vi "SSL_Certification.vi"(8 "error in (no error)":errorcluster, 11 "DUT":string) -> (0 "error in (out)":errorcluster, 2 "Result":string)   [LabVIEW 2024, in "SSL_Certification.lvlib"]
doc: "This template is for the Queued Message Handler design pattern.\n\nThe Event Handling Loop generates messages based on user interface actions.\n\nThe Message Handling Loop processes messages generated by the Event Handling Loop, or by other messages. The messages are string values, so new messages can be added easily to the Message Cases case structure in the Message Handling Loop. Each message cluster can also provide an optional value for Message Data, which is a variant that can be converted to whatever message-specific data is required."
uses:
  SSL_Certification.lvlib
  support/Neoway_ctrl.ctl
  controls/Neoway UI Data.ctl
  PrivateControls/FGV_Queue_Control.ctl
  <vilib>/Utility/error.llb/Trim Whitespace One-Sided.vi
  <vilib>/Utility/error.llb/Error Cluster From Error Code.vi
  <vilib>/ErrorRing/Error Ring.xnode
  support/Message Queue/Neoway Message Queue.lvlib
  support/User Event - Stop/72-13360 User Event - Stop.lvlib
  Launcher/Launcher_DTU.lvlib
panel:
  out "Timer":i32
  in  "Neoway Flashing":T1
  in  "Config":string
  in  "Read_Res":bool
  in  "Read_Current":bool
  in  "Read_File":bool
  in  "Flash":bool
  out "queue name 2":string
  out "queue name":string
  out "Display <Replace Me>":string
  in  "Output":bool
  in  "Init_Neoway":bool
  in  "Exit":bool
  # "OKAY,River"
  # "These controls have associated \"Value Changed\" events configured in the Event Structure on the diagram.\n\nReplace them (and reconfigure the Event Structure) with the controls you need for your application."
  # "This template is for the Queued Message Handler design pattern.\n\nSee the block diagram for more information on how to use this template."
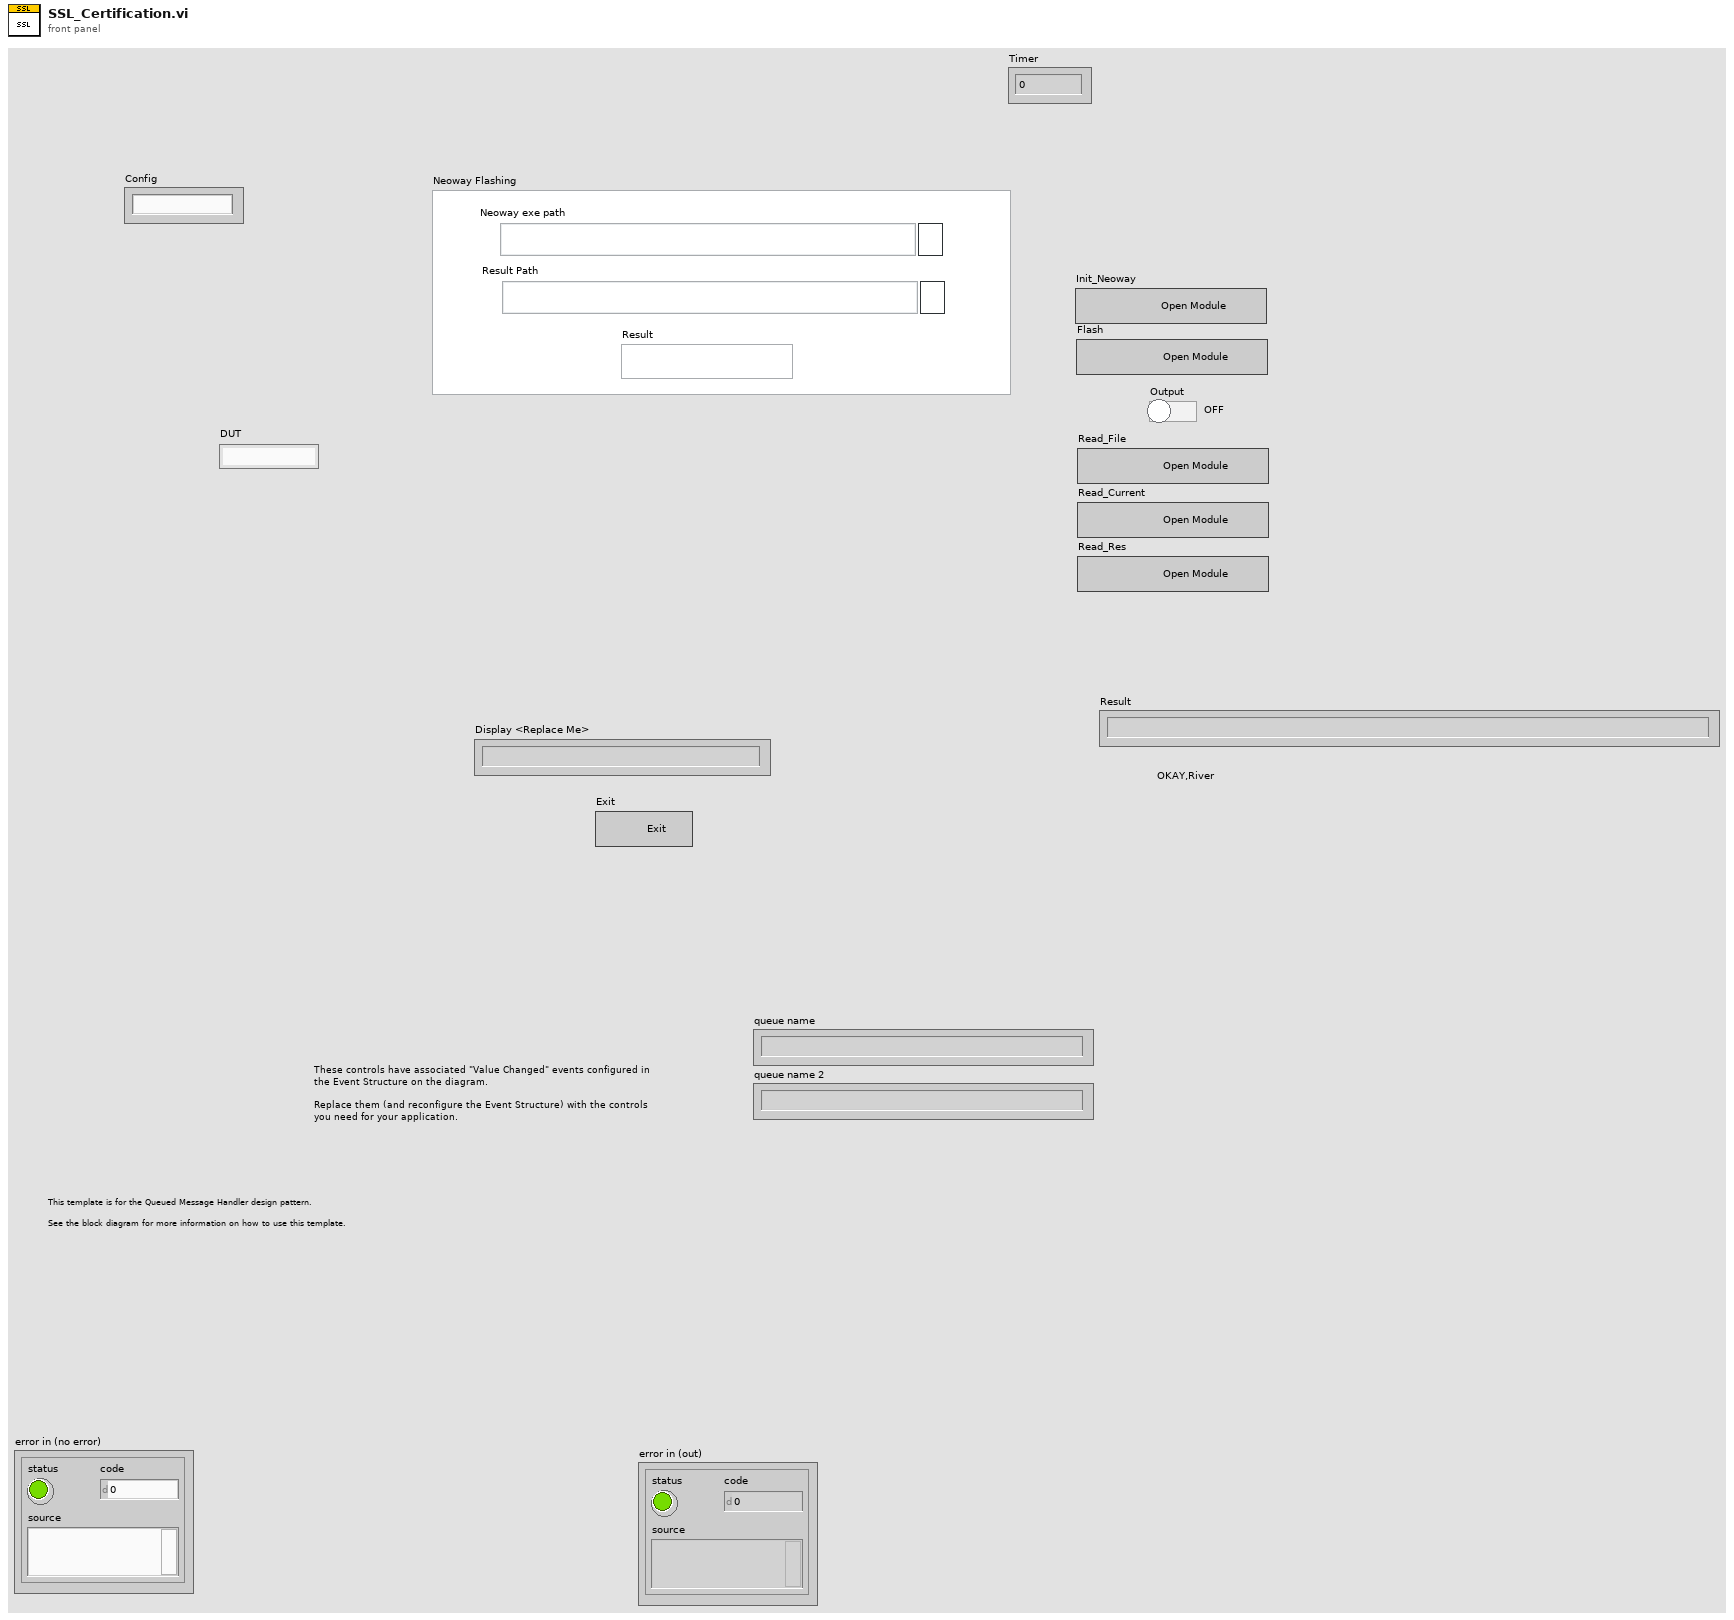
[diagram p1: front panel]
types:
  T1 = typedef "SSL_Certification.lvlib/Neoway_ctrl.ctl" = cluster{"Neoway exe path":path, "Result Path":path, "Result":string}
  T2 = typedef "SSL_Certification.lvlib/Neoway UI Data.ctl" = cluster{"DUT":string, "Neoway_Q":refnum<queue>, "notifier out":refnum<notifier>, "Config":string, "Neoway Flashing":T1, "Bat file path":path, "Exe path":string, "Flash path":string, "Result":string, "Timer":u32}
  T3 = typedef "SSL_Certification.lvlib/FGV_Queue_Control.ctl" = enum16{"Release", "Get", "Set"}
  T4 = typedef "SSL_Certification.lvlib/Neoway Message Queue.lvlib/All Message Queues.ctl" = cluster{"UI":refnum<queue>, "QSM":refnum<queue>}
  T5 = cluster{"Message":string, "Message Data":variant}
  T6 = enum16{"Read", "Write", "All_sections", "All_values", "Remove key&section"}
  T7 = enum16{"open", "replace", "create", "open or create", "replace or create", "replace or create with confirmation"}
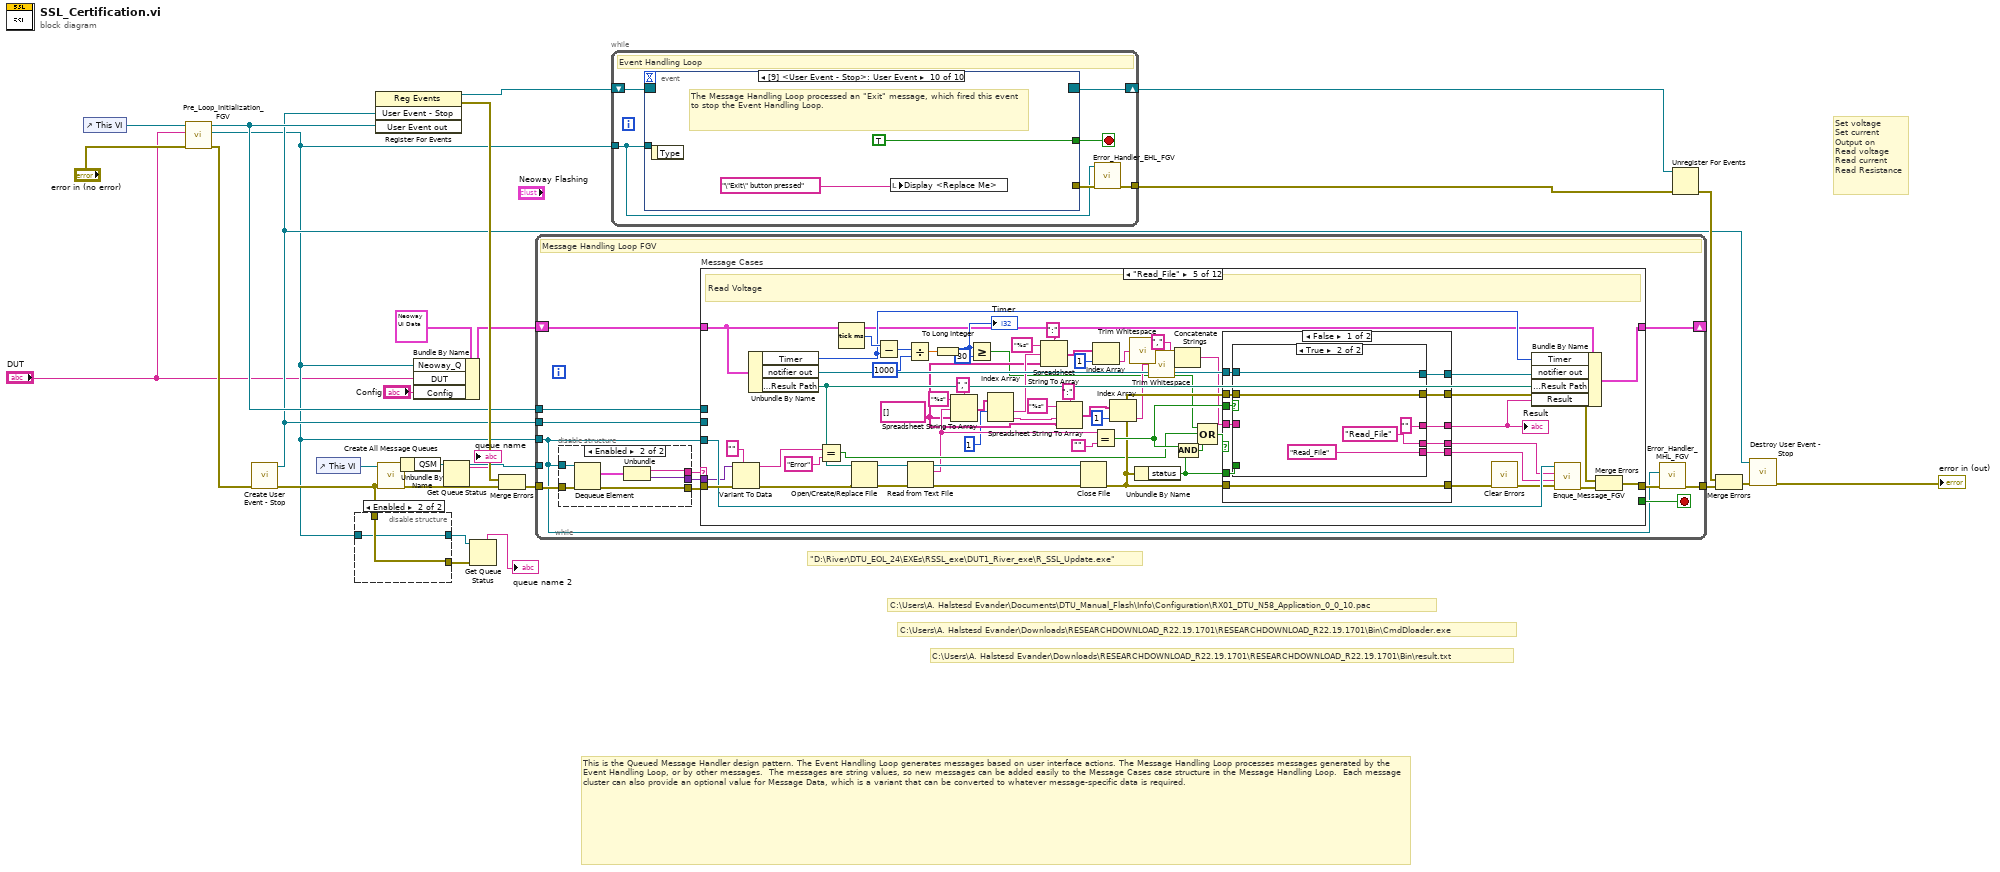
[diagram p0: block diagram]
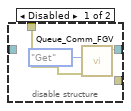
[diagram p2: hidden frame]
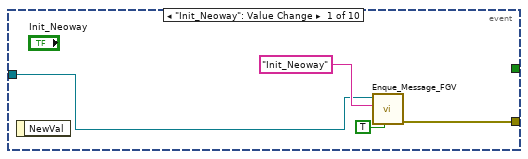
[diagram p3: hidden frame]
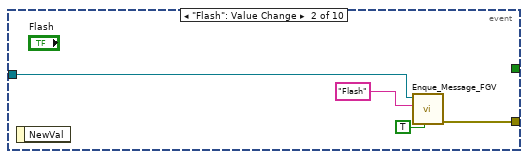
[diagram p4: hidden frame]
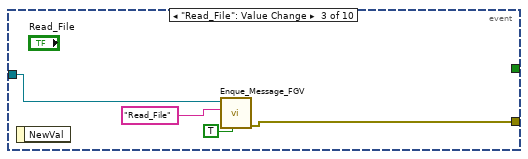
[diagram p5: hidden frame]
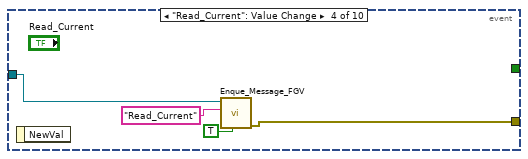
[diagram p6: hidden frame]
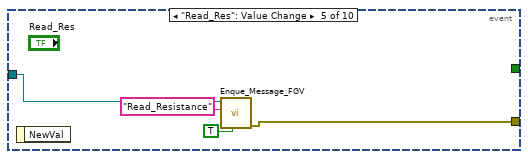
[diagram p7: hidden frame]
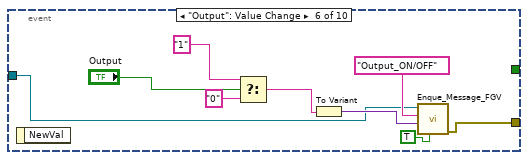
[diagram p8: hidden frame]
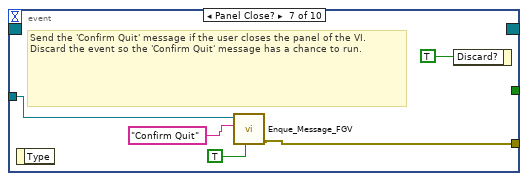
[diagram p9: hidden frame]
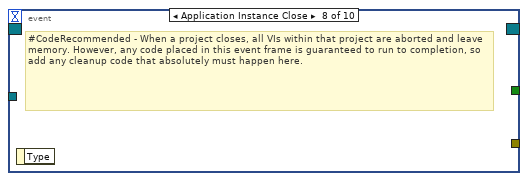
[diagram p10: hidden frame]
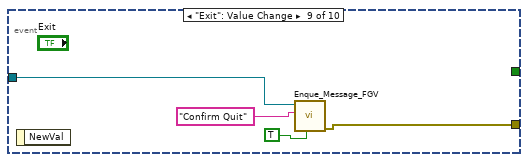
[diagram p11: hidden frame]
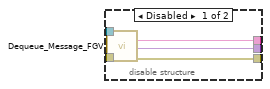
[diagram p12: hidden frame]
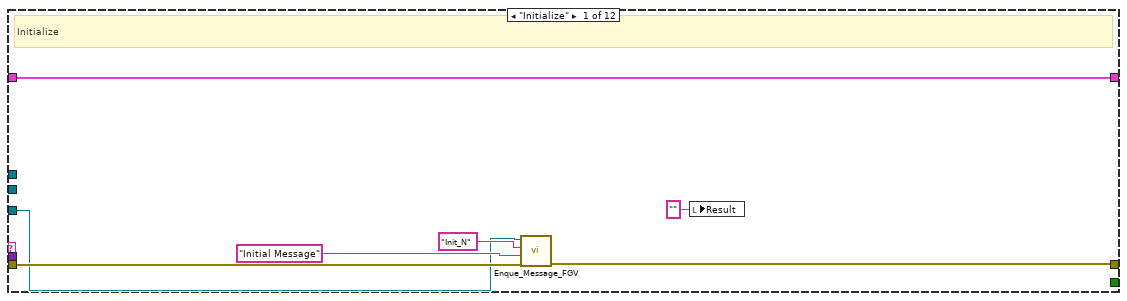
[diagram p13: hidden frame]
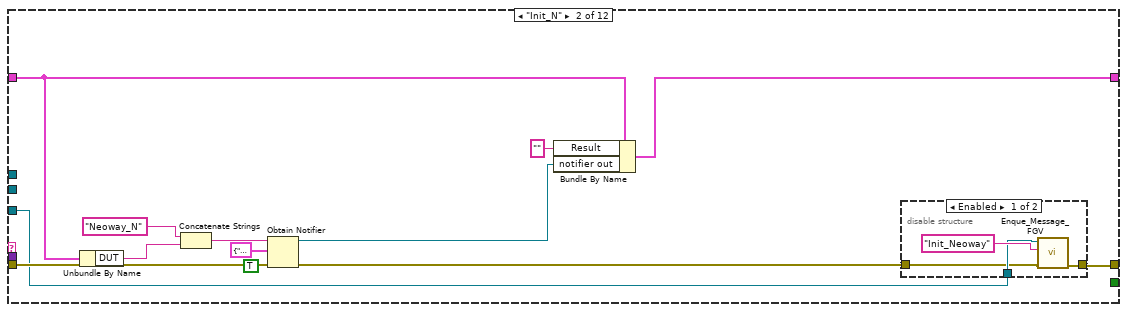
[diagram p14: hidden frame]
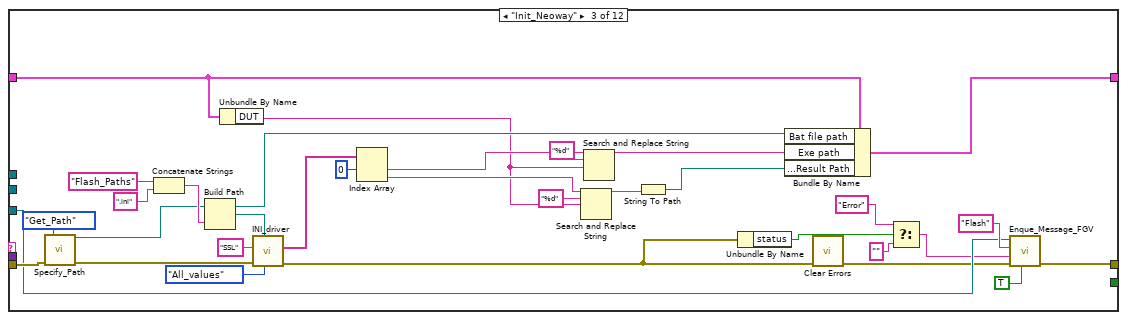
[diagram p16: hidden frame]
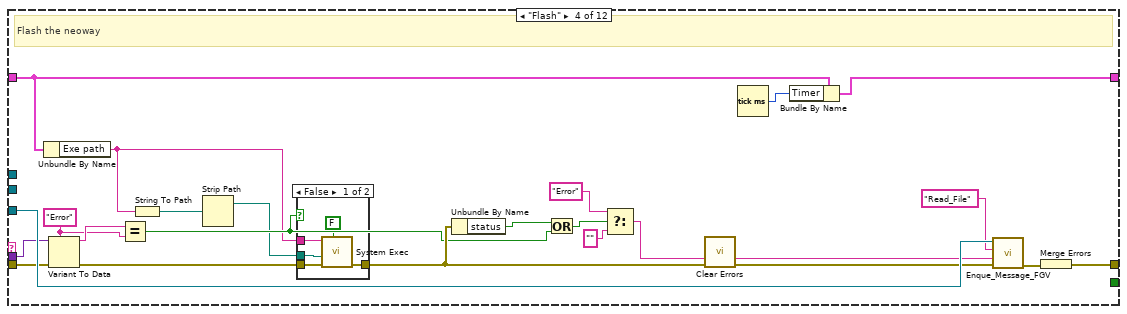
[diagram p17: hidden frame]
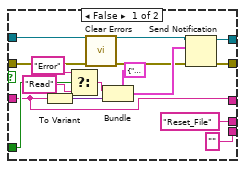
[diagram p19: hidden frame]
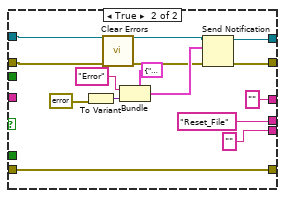
[diagram p20: hidden frame]
diagram:
  # "\"D:\\River\\DTU_EOL_24\\EXEs\\RSSL_exe\\DUT1_River_exe\\R_SSL_Update.exe\""
  # "C:\\Users\\A. Halstesd Evander\\Downloads\\RESEARCHDOWNLOAD_R22.19.1701\\RESEARCHDOWNLOAD_R22.19.1701\\Bin\\result.txt"
  # "C:\\Users\\A. Halstesd Evander\\Downloads\\RESEARCHDOWNLOAD_R22.19.1701\\RESEARCHDOWNLOAD_R22.19.1701\\Bin\\CmdDloader.exe"
  # "C:\\Users\\A. Halstesd Evander\\Documents\\DTU_Manual_Flash\\Info\\Configuration\\RX01_DTU_N58_Application_0_0_10.pac"
  # "Set voltage\nSet current\nOutput on\nRead voltage \nRead current\nRead Resistance"
  # "This is the Queued Message Handler design pattern. The Event Handling Loop generates messages based on user interface actions. The Message Handling Loop processes messages generated by the Event Handling Loop, or by other messages.  The messages are string values, so new messages can be added easily to the Message Cases case structure in the Message Handling Loop.  Each message cluster can also provide an optional value for Message Data, which is a variant that can be converted to whatever message-specific data is required."
  n1 = control-ref of="This VI"() -> (w17:refnum<vi>)
  n2 = call "Pre_Loop_Initialization_FGV.vi"("error in (no error)"="error in (no error)", "DUT"="DUT", "VI in"=w17) -> ("error out"=w15:errorcluster, "queue out"=w3:refnum<queue>, "User Event out"=w7:refnum<user-event>)  [unwired: 6 in]
  n3 = call "Create User Event - Stop.vi"("error in (no error)"=w15) -> ("error out"=w10:errorcluster, "User Event - Stop"=w6:refnum<user-event>)  [unwired: 9 in]
  n4 = control-ref of="This VI"() -> (w13:refnum<vi>)
  n5 = disable-structure shown="Enabled" {
    disable-tunnel: w10 -> [w32 w34]
    disable-tunnel: [w30 w33] -> w9
    disable-tunnel: [_ w34] -> w5
    disable-tunnel: w3 -> [_ w33]
    frame Disabled {
      n6 = call "Queue_Comm_FGV.vi"("error in (no error)"=w32, "Enum"=FGV_Queue_Control."Get") -> ("queue Out"=w30:refnum<queue>)  [unwired: 8 in, 1 out]
    }
    frame Enabled {
    }
  }
  n7 = register-events(w6, w7) -> (reference out=w20:refnum<event-registration>, error out=w18:errorcluster)  [unwired: 2 in]
  n8 = call "Create All Message Queues.vi"("error in (no error)"=w10, "This VI"=w13) -> ("error out"=w29:errorcluster, "Message Queues out"=w28:T4)  [unwired: 8 in]
  n9 = Unbundle By Name(w28) -> ("QSM"=w26:refnum<queue>)
  n10 = Bundle By Name(cluster=T2 {"DUT"="", "Neoway_Q"=refnum, "notifier out"=refnum, "Config"="", "Neoway Flashing"={"Neoway exe path"=path "", "Result Path"=path "", "Result"=""}, "Bat file path"=path "", "Exe path"="", "Flash path"="", "Result"="", "Timer"=0} ("Data Cluster"), "Neoway_Q"=w3, "DUT"="DUT", "Config"="Config") -> (w4:T2)
  n11 = Get Queue Status(queue=w26) -> (queue out=w12:refnum<queue>, queue name=→"queue name":string)  [unwired: 2 in, 6 out]
  n12 = Get Queue Status(queue=w9, error in (no error)=w5) -> (queue name=→"queue name 2":string)  [unwired: 1 in, 7 out]
  n13 = Merge Errors(w18, w29) -> (w19:errorcluster)
  n14 = while {
    tunnel: w12 -> [_]
    shift-right: [w45] -> _
    shift-left: w4 -> [w46]
    tunnel: w7 -> [w43]
    tunnel: w19 -> [w42]
    tunnel: [w37] -> w27
    tunnel: w6 -> [w36]
    tunnel: w3 -> [w35]
    stop <- w44 stop-if-true
    # "Message Handling Loop FGV"
    n15 = disable-structure shown="Enabled" {
      disable-tunnel: w42 -> [w50 w56]
      disable-tunnel: [w49 w54] -> w41
      disable-tunnel: [w48 w51] -> w40
      disable-tunnel: [w47 w52] -> w39
      disable-tunnel: w35 -> [_ w55]
      frame Disabled {
        n16 = call "Dequeue_Message_FGV.vi"("error in (no error)"=w50) -> ("error out"=w49:errorcluster, "Message Data"=w48:variant, "Message"=w47:string)  [unwired: 8 in]
      }
      frame Enabled {
        n17 = Dequeue Element(queue=w55, error in (no error)=w56) -> (element=w53:T5, error out=w54:errorcluster)  [unwired: 1 in, 2 out]
        n18 = Unbundle(w53) -> ("Message"=w52:string, "Message Data"=w51:variant)
      }
    }
    n19 = case "Message Cases" shown="\"Read_File\"" w39 {
      selector: w39 -> [_ _ _ _ _ _ _ _ _ _ _ w313]
      tunnel: w41 -> [w59 w76 w113 w133 w203 w263 w273 w282 w291 w296 w304 _]
      tunnel: [w62 w65 w89 w136 w199 w250 w265 w280 w293 w294 w297 w314] -> w38
      tunnel: w46 -> [w63 w74 w98 w132 w143 w262 w274 w281 w288 w295 w299 w315]
      tunnel: [w63 w69 w103 w115 w201 w262 w274 w281 w288 w295 w299 w315] -> w45
      tunnel: [_ _ _ _ _ _ _ _ _ _ TRUE _] -> w44
      tunnel: w40 -> [_ _ _ w123 w198 _ w272 _ _ _ w306 _]
      tunnel: w43 -> [_ _ _ _ _ _ _ _ _ _ w307 _]
      tunnel: w36 -> [_ _ _ _ _ _ _ _ _ _ w302 _]
      tunnel: w35 -> [w58 w67 w88 w134 w200 w249 w264 w275 w286 _ w298 _]
      frame "Initialize" {
        # "Initialize"
        n20 = call "Enque_Message_FGV.vi"("error in (no error)"=w59, "Message Data"="Initial Message" ("Initial Message"), "Message"="Init_N", "queue in"=w58) -> ("error out"=w62:errorcluster)  [unwired: 7 in]
        n21 = local write "Result"("" ("Result")) -> ()
      }
      frame "Init_N" {
        n22 = Unbundle By Name(w74) -> ("DUT"=w73:string)
        n23 = Concatenate Strings("Neoway_N", w73) -> (w72:string)
        n24 = Obtain Notifier(name (unnamed)=w72, notification data type=T5 {"Message"="", "Message Data"=variant} ("notification"), create if not found? (T)=TRUE, error in (no error)=w76) -> (notifier out=w68:refnum<notifier>, error out=w66:errorcluster)  [unwired: 1 out]
        n25 = Bundle By Name(cluster=w74, "Result"="", "notifier out"=w68) -> (w69:T2)
        n26 = disable-structure shown="Enabled" {
          disable-tunnel: w67 -> [w79 _]
          disable-tunnel: w66 -> [w78 w81]
          disable-tunnel: [w77 w81] -> w65
          frame Enabled {
            n27 = call "Enque_Message_FGV.vi"("error in (no error)"=w78, "Message"="Init_Neoway", "queue in"=w79) -> ("error out"=w77:errorcluster)  [unwired: 8 in]
          }
          frame Disabled {
          }
        }
      }
      frame "Init_Neoway" {
        n28 = call "Specify_Path.vi"("Path_Enum"=enum16{"Find_Path", "Get_Path"}."Get_Path", "error in (no error)"=w113) -> ("Configurations"=w101:path, "error out"=w108:errorcluster)  [unwired: 6 in, 6 out]
        n29 = Concatenate Strings("Flash_Paths" ("string"), ".ini" ("string")) -> (w110:string)
        n30 = Build Path(base path=w101, name or relative path=w110) -> (appended path=w109:path)
        n31 = Unbundle By Name(w98) -> ("DUT"=w94:string)
        n32 = call "INI_driver.vi"("Enum"=T6."All_values", "instrument file path"=w109, "error in (no error)"=w108, "Section"="SSL") -> ("error out"=w84:errorcluster, "Values out"=w106:string[])  [unwired: 4 in, 2 out]
        n33 = Index Array(array=w106, index #1=0 ("index")) -> (element #1=w100:string, element #2=w95:string)  [unwired: 1 in]
        n34 = Search and Replace String(input string=w95, search string="%d", replace string=w94) -> (result string=w93:string)  [unwired: 5 in, 3 out]
        n35 = Search and Replace String(input string=w100, search string="%d", replace string=w94) -> (result string=w97:string)  [unwired: 5 in, 3 out]
        n36 = String To Path(string=w93) -> (path=w92:path)
        n37 = Unbundle By Name(w84) -> ("status"=w86:bool)
        n38 = Bundle By Name(cluster=w98, "Bat file path"=w101, "Exe path"=w97, "Neoway Flashing.Result Path"=w92) -> (w103:T2)
        n39 = call <vilib>:"Clear Errors.vi"("error in (no error)"=w84) -> ("error out"=w82:errorcluster)  [unwired: 5 in, 1 out]
        n40 = Select(t="Error" ("\"Do Something\" button pressed"), s=w86, f="" ("\"Do Something\" button pressed")) -> (s? t:f=w83:string)
        n41 = call "Enque_Message_FGV.vi"("Priority"=TRUE ("Priority Message? (F)"), "error in (no error)"=w82, "Message Data"=w83, "Message"="Flash", "queue in"=w88) -> ("error out"=w89:errorcluster)  [unwired: 6 in]
      }
      frame "Flash" {
        w120 = "Error" ("Message")
        # "Flash the neoway"
        n42 = Unbundle By Name(w132) -> ("Exe path"=w118:string)
        n43 = Variant To Data(error in=w133, type=w120, Variant=w123) -> (data=w121:string, error out=w124:errorcluster)
        n44 = Equal?(x=w121, y=w120) -> (x = y?=w119:bool)
        n45 = String To Path(string=w118) -> (path=w117:path)
        n46 = Strip Path(path=w117) -> (stripped path=w116:path)  [unwired: 1 out]
        n47 = case shown="False" w119 {
          tunnel: w118 -> [w141 _]
          tunnel: [w140 w142] -> w131
          tunnel: w124 -> [w139 w142]
          tunnel: w116 -> [w137 _]
          frame False {
            n48 = call <vilib>:"System Exec.vi"("wait until completion? (T)"=FALSE, "error in (no error)"=w139, "working directory"=w137, "command line"=w141) -> ("error out"=w140:errorcluster)  [unwired: 4 in, 3 out]
          }
          frame True {
          }
        }
        n49 = Unbundle By Name(w131) -> ("status"=w128:bool)
        n50 = Or(x=w128, y=w119) -> (x .or. y?=w122:bool)
        n51 = Select(t="Error" ("\"Do Something\" button pressed"), s=w122, f="" ("\"Do Something\" button pressed")) -> (s? t:f=w126:string)
        n52 = call <vilib>:"Clear Errors.vi"("error in (no error)"=w131) -> ("error out"=w125:errorcluster)  [unwired: 5 in, 1 out]
        n53 = Tick Count (ms)() -> (millisecond timer value=w114:u32)
        n54 = Bundle By Name(cluster=w132, "Timer"=w114) -> (w115:T2)
        n55 = call "Enque_Message_FGV.vi"("error in (no error)"=w125, "Message Data"=w126, "Message"="Read_File", "queue in"=w134) -> ("error out"=w135:errorcluster)  [unwired: 7 in]
        n56 = Merge Errors(w135) -> (w136:errorcluster)
      }
      frame "Read_File" {
        w165 = string[] []
        # "Read Voltage"
        n57 = Variant To Data(error in=w203, type="", Variant=w198) -> (data=w195:string, error out=w194:errorcluster)
        n58 = Unbundle By Name(w143) -> ("Timer"=w149:u32, "notifier out"=w185:refnum<notifier>, "Neoway Flashing.Result Path"=w188:path)
        n59 = Equal?(x=w195, y="Error" ("\"Do Something\" button pressed")) -> (x = y?=w177:bool)
        n60 = Tick Count (ms)() -> (millisecond timer value=w155:u32)
        n61 = Open/Create/Replace File(file path (use dialog)=w188, error in=w194) -> (refnum out=w191:refnum<file>, error out=w193:errorcluster)  [unwired: 4 in, 1 out]
        n62 = Subtract(x=w155, y=w149) -> (x-y=w154:u32)
        n63 = Divide(x=w154, y=u32 1000) -> (x/y=w152:dbl)
        n64 = Read from Text File(file (use dialog)=w191, error in=w193) -> (refnum out=w189:refnum<file>, text=w174:string, error out=w192:errorcluster)  [unwired: 2 in, 1 out]
        n65 = To Long Integer(number=w152) -> (32bit integer=w148:i32)
        "Timer" <- w148
        n66 = Spreadsheet String To Array(delimiter (Tab)=",", format string="%s", spreadsheet string=w174, array type (2D Dbl)=w165) -> (array=w171:string[])
        n67 = Greater Or Equal?(x=w148, y=30) -> (x >= y?=w150:bool)
        n68 = Index Array(array=w171, index #1=1 ("index")) -> (element #1=w166:string, element #2=w164:string)  [unwired: 1 in]
        n69 = Spreadsheet String To Array(delimiter (Tab)=":", format string="%s", spreadsheet string=w166, array type (2D Dbl)=w165) -> (array=w163:string[])
        n70 = Spreadsheet String To Array(delimiter (Tab)=":", format string="%s", spreadsheet string=w164, array type (2D Dbl)=w165) -> (array=w160:string[])
        n71 = Close File(refnum=w189, error in=w192) -> (error out=w179:errorcluster)  [unwired: 1 out]
        n72 = Equal?(x=w174, y="") -> (x = y?=w182:bool)
        n73 = Index Array(array=w163, index=1) -> (element=w159:string)
        n74 = Index Array(array=w160, index=1) -> (element=w157:string)
        n75 = call <vilib>:"Trim Whitespace.vi"("string"=w159) -> ("trimmed string"=w145:string)  [unwired: 1 in]
        n76 = Unbundle By Name(w179) -> ("status"=w183:bool)
        n77 = call <vilib>:"Trim Whitespace.vi"("string"=w157) -> ("trimmed string"=w144:string)  [unwired: 1 in]
        n78 = Concatenate Strings(w145, "," ("string"), w144) -> (w156:string)
        n79 = Compound Arithmetic op=AND(w182, w183) -> (w176:bool)
        n80 = Compound Arithmetic op=OR(w150, w177, w176) -> (w175:bool)
        n81 = case shown="False" w175 {
          tunnel: w179 -> [w214 w240]
          tunnel: [w213 w241] -> w186
          tunnel: w185 -> [w212 w243]
          tunnel: [w211 w242] -> w184
          tunnel: w156 -> [w210 _]
          tunnel: w183 -> [w209 _]
          tunnel: w182 -> [w208 _]
          tunnel: [w207 "Reset_File" ("Message")] -> w181
          tunnel: [w206 "" ("\"Do Something\" button pressed")] -> w180
          tunnel: w179 -> [w205 w248]
          tunnel: [w205 w248] -> w178
          tunnel: [w204 ""] -> w147
          frame False {
            n82 = case shown="True" w208 {
              tunnel: w214 -> [w223 w234]
              tunnel: [w221 w234] -> w213
              tunnel: w212 -> [w220 w233]
              tunnel: [w219 w233] -> w211
              tunnel: w210 -> [w215 _]
              tunnel: w209 -> [w218 _]
              tunnel: ["Reset_File" ("Message") "Read_File" ("Message")] -> w207
              tunnel: ["" ("\"Do Something\" button pressed") "Read_File" ("\"Do Something\" button pressed")] -> w206
              tunnel: [w215 ""] -> w204
              frame False {
                n83 = To Variant(anything=w215) -> (Variant=w228:variant)
                n84 = Select(t="Error" ("f"), s=w218, f="Read" ("Message")) -> (s? t:f=w229:string)
                n85 = call <vilib>:"Clear Errors.vi"("error in (no error)"=w223) -> ("error out"=w222:errorcluster)  [unwired: 5 in, 1 out]
                n86 = Bundle(cluster=T5 {"Message"="", "Message Data"=variant} ("notification"), "Message"=w229, "Message Data"=w228) -> (w227:T5)
                n87 = Send Notification(notification=w227, notifier=w220, error in (no error)=w222) -> (notifier out=w219:refnum<notifier>, error out=w221:errorcluster)
              }
              frame True {
              }
            }
          }
          frame True {
            n88 = To Variant(anything=errorcluster {"status"=TRUE, "code"=0, "source"="Error at N58 Flashing"} ("error constant")) -> (Variant=w247:variant)
            n89 = call <vilib>:"Clear Errors.vi"("error in (no error)"=w240) -> ("error out"=w244:errorcluster)  [unwired: 5 in, 1 out]
            n90 = Bundle(cluster=T5 {"Message"="", "Message Data"=variant} ("notification"), "Message"="Error" ("f"), "Message Data"=w247) -> (w246:T5)
            n91 = Send Notification(notification=w246, notifier=w243, error in (no error)=w244) -> (notifier out=w242:refnum<notifier>, error out=w241:errorcluster)
          }
        }
        "Result" <- w147
        n92 = call <vilib>:"Clear Errors.vi"("error in (no error)"=w178) -> ("error out"=w187:errorcluster)  [unwired: 5 in, 1 out]
        n93 = Bundle By Name(cluster=w143, "Timer"=w149, "notifier out"=w184, "Neoway Flashing.Result Path"=w188, "Result"=w147) -> (w201:T2)
        n94 = call "Enque_Message_FGV.vi"("error in (no error)"=w187, "Message Data"=w180, "Message"=w181, "queue in"=w200) -> ("error out"=w202:errorcluster)  [unwired: 7 in]
        n95 = Merge Errors(w186, w202) -> (w199:errorcluster)
      }
      frame "Reset_File" {
        n96 = Unbundle By Name(w262) -> ("Neoway Flashing.Result Path"=w260:path)  [unwired: 1 out]
        n97 = Open/Create/Replace File(file path (use dialog)=w260, error in=w263, operation (0:open)=T7."replace") -> (refnum out=w257:refnum<file>, error out=w261:errorcluster)  [unwired: 3 in, 1 out]
        n98 = Read from Text File(file (use dialog)=w257, error in=w261) -> (refnum out=w254:refnum<file>, text=w255:string, error out=w258:errorcluster)  [unwired: 2 in, 1 out]
        n99 = Equal?(x=w255, y="") -> ()  [unwired: 1 out]
        n100 = Close File(refnum=w254, error in=w258) -> (error out=w251:errorcluster)  [unwired: 1 out]
        n101 = call "Enque_Message_FGV.vi"("error in (no error)"=w251, "Message Data"="Resetted Flash file" ("\"Do Something\" button pressed"), "Message"="Update Display", "queue in"=w249) -> ("error out"=w250:errorcluster)  [unwired: 7 in]
      }
      frame "Update Display" {
        # "#CodeRecommended - If you wish to decouple the Message Handling Loop from your user interface, consider creating User Events (like the \"Stop\" event in this VI) to message the Event Handling Loop whenever the user interface needs updating."
        # "Update Display - Convert the message data to a string to display in the Data Display indicator."
        n102 = Variant To Data(error in=w273, type="", Variant=w272) -> (data=→"Display <Replace Me>":string, error out=w270:errorcluster)
        n103 = call <vilib>:"Clear Errors.vi"("error in (no error)"=w270) -> ("error out"=w268:errorcluster)  [unwired: 5 in, 1 out]
        n104 = Merge Errors(w268) -> (w266:errorcluster)
        n105 = call "Enque_Message_FGV.vi"("error in (no error)"=w266, "Message"="Confirm Quit", "queue in"=w264) -> ("error out"=w265:errorcluster)  [unwired: 8 in]
      }
      frame "Error" {
        # "Error - Display an error dialog. This message is sent by the \"Error Handler\" VIs at the end of other loops in this application."
        n106 = call <vilib>:"Clear Errors.vi"("error in (no error)"=w282) -> ("error out"=w277:errorcluster)  [unwired: 5 in, 1 out]
        n107 = call "Enque_Message_FGV.vi"("Priority"=TRUE ("Priority Message? (F)"), "error in (no error)"=w277, "Message"="Confirm Quit", "queue in"=w275) -> ("error out"=w276:errorcluster)  [unwired: 7 in]
        n108 = Merge Errors(w276) -> (w280:errorcluster)
      }
      frame "Confirm Quit" {
        # "Confirm Quit - Message that can confirm whether or not the user wants to exit the application."
        n109 = Unbundle By Name(w288) -> ("notifier out"=w284:refnum<notifier>)
        n110 = Release Notifier(notifier=w284, force destroy? (F)=TRUE, error in (no error)=w291) -> (error out=w285:errorcluster)  [unwired: 2 out]
        n111 = call <vilib>:"Clear Errors.vi"("error in (no error)"=w285) -> ("error out"=w287:errorcluster)  [unwired: 5 in, 1 out]
        n112 = call "Enque_Message_FGV.vi"("Priority"=TRUE ("Priority Message? (F)"), "error in (no error)"=w287, "Message"="Exit", "queue in"=w286) -> ("error out"=w292:errorcluster)  [unwired: 7 in]
        n113 = Merge Errors(w292) -> (w293:errorcluster)
      }
      frame "---Copy This Frame---" {
        # "Duplicate this frame when creating new messages.  Change this comment in the duplicated frame to describe this message."
        n114 = Merge Errors(w296) -> (w294:errorcluster)
      }
      frame "Exit" {
        # "Stop the VI"
        # "Release the message queue reference"
        # "Exit - Exit the application."
        n115 = disable-structure shown="Enabled" {
          disable-tunnel: w306 -> [w310 _]
          frame Disabled {
            n116 = Variant To Data(type=errorcluster {"status"=FALSE, "code"=0, "source"=""} ("error constant"), Variant=w310) -> (data=w311:errorcluster)  [unwired: 1 in, 1 out]
            n117 = call <vilib>:"Simple Error Handler.vi"("error in (no error)"=w311) -> ()  [unwired: 4 in, 5 out]
          }
          frame Enabled {
          }
        }
        n118 = call "Queue_Comm_FGV.vi"("error in (no error)"=w304, "Enum"=FGV_Queue_Control."Release", "queue in"=w298) -> ("error Out"=w303:errorcluster)  [unwired: 7 in, 1 out]
        n119 = call "Fire User Event - Stop.vi"("User Event - Stop"=w302) -> ("error out"=w300:errorcluster)  [unwired: 10 in]
        n120 = call "Fire User Event - Stop.vi"("User Event - Stop"=w307) -> ("error out"=w301:errorcluster)  [unwired: 10 in]
        n121 = Merge Errors(w301, w300, w303) -> (w308:errorcluster)
        n122 = call <vilib>:"Clear Errors.vi"("error in (no error)"=w308) -> ("error out"=w297:errorcluster)  [unwired: 5 in, 1 out]
      }
      frame Default {
        # "'Default' case only runs if there is a message that isn't defined in any of the other cases.  Output a programming error."
        n123 = xnode "Error Ring"("parameter 0"=w313) -> ("error out"=w314:errorcluster)
      }
    }
    n124 = call "Error_Handler_MHL_FGV.vi"("error in (no error)"=w38, "queue in"=w35) -> ("error Out"=w37:errorcluster)  [unwired: 9 in]
  }
  n125 = while {
    shift-right: [w327] -> w23
    shift-left: w20 -> [w328]
    tunnel: [w324] -> w21
    tunnel: w3 -> [w323]
    stop <- w326 stop-if-true
    # "Event Handling Loop"
    n126 = event shown="[9] <User Event - Stop>: User Event" {
      selector: w328 -> [_ _ _ _ _ _ _ _ _ _]
      dyn-events: [_ _ _ _ _ _ _ _ _ _] -> w327
      timeout: _ -> [_ _ _ _ _ _ _ _ _ _]
      tunnel: [_ _ _ _ _ _ _ _ _ TRUE ("Discard?")] -> w326
      tunnel: [w331 w335 w339 w343 w347 w355 w361 _ w366 _] -> w325
      tunnel: w323 -> [w329 w333 w337 w341 w345 w349 w358 _ w363 _]
      event "Init_Neoway": Value Change {
        n127 = event-data() -> ()  [unwired: 1 in, 1 out]
        n128 = call "Enque_Message_FGV.vi"("Priority"=TRUE ("Priority Message? (F)"), "Message"="Init_Neoway", "queue in"=w329) -> ("error out"=w331:errorcluster)  [unwired: 8 in]
      }
      event "Flash": Value Change {
        n129 = event-data() -> ()  [unwired: 1 in, 1 out]
        n130 = call "Enque_Message_FGV.vi"("Priority"=TRUE ("Priority Message? (F)"), "Message"="Flash", "queue in"=w333) -> ("error out"=w335:errorcluster)  [unwired: 8 in]
      }
      event "Read_File": Value Change {
        n131 = event-data() -> ()  [unwired: 1 in, 1 out]
        n132 = call "Enque_Message_FGV.vi"("Priority"=TRUE ("Priority Message? (F)"), "Message"="Read_File", "queue in"=w337) -> ("error out"=w339:errorcluster)  [unwired: 8 in]
      }
      event "Read_Current": Value Change {
        n133 = event-data() -> ()  [unwired: 1 in, 1 out]
        n134 = call "Enque_Message_FGV.vi"("Priority"=TRUE ("Priority Message? (F)"), "Message"="Read_Current", "queue in"=w341) -> ("error out"=w343:errorcluster)  [unwired: 8 in]
      }
      event "Read_Res": Value Change {
        n135 = event-data() -> ()  [unwired: 1 in, 1 out]
        n136 = call "Enque_Message_FGV.vi"("Priority"=TRUE ("Priority Message? (F)"), "Message"="Read_Resistance", "queue in"=w345) -> ("error out"=w347:errorcluster)  [unwired: 8 in]
      }
      event "Output": Value Change {
        n137 = event-data() -> ()  [unwired: 1 in, 1 out]
        n138 = Select(t="1", s="Output", f="0") -> (s? t:f=w351:string)
        n139 = To Variant(anything=w351) -> (Variant=w350:variant)
        n140 = call "Enque_Message_FGV.vi"("Priority"=TRUE ("Priority Message? (F)"), "Message Data"=w350, "Message"="Output_ON/OFF", "queue in"=w349) -> ("error out"=w355:errorcluster)  [unwired: 7 in]
      }
      event Panel Close? {
        # "Send the 'Confirm Quit' message if the user closes the panel of the VI. Discard the event so the 'Confirm Quit' message has a chance to run."
        n141 = event-data() -> ()  [unwired: 1 in, 1 out]
        n142 = call "Enque_Message_FGV.vi"("Priority"=TRUE ("Priority Message? (F)"), "Message"="Confirm Quit", "queue in"=w358) -> ("error out"=w361:errorcluster)  [unwired: 8 in]
        n143 = event-data("Discard?"=TRUE) -> ()  [unwired: 1 in, 1 out]
      }
      event Application Instance Close {
        # "#CodeRecommended - When a project closes, all VIs within that project are aborted and leave memory. However, any code placed in this event frame is guaranteed to run to completion, so add any cleanup code that absolutely must happen here."
        n144 = event-data() -> ()  [unwired: 1 in, 1 out]
      }
      event "Exit": Value Change {
        n145 = event-data() -> ()  [unwired: 1 in, 1 out]
        n146 = call "Enque_Message_FGV.vi"("Priority"=TRUE ("Priority Message? (F)"), "Message"="Confirm Quit", "queue in"=w363) -> ("error out"=w366:errorcluster)  [unwired: 8 in]
      }
      event User Event {
        # "The Message Handling Loop processed an \"Exit\" message, which fired this event to stop the Event Handling Loop."
        n147 = event-data() -> ()  [unwired: 1 in, 1 out]
        n148 = local write "Display <Replace Me>"("\"Exit\" button pressed" ("VI Stopped")) -> ()
      }
    }
    n149 = call "Error_Handler_EHL_FGV.vi"("error in (no error)"=w325, "queue in"=w323) -> ("error Out"=w324:errorcluster)  [unwired: 9 in]
  }
  n150 = Unregister For Events(event registration refnum=w23, error in=w21) -> (error out=w24:errorcluster)
  n151 = Merge Errors(w24, w27) -> (w25:errorcluster)
  n152 = call "Destroy User Event - Stop.vi"("error in (no error)"=w25, "User Event - Stop"=w6) -> ("error out"=→"error in (out)":errorcluster)  [unwired: 9 in]
